vi "加标回收启动对话框.vi"(11 "测试模式":enum16{"水样测试", "平行样测试", "加标回收", "集成干预测试"}(ring)) -> (1 "流程参数":T2, 2 "启动参数":T3, 3 "check ？":bool)   [LabVIEW 2016, in "质控单元V2.lvlib"]
panel:
  in  "静态加标设置":T1
  in  "采配水":bool=TRUE
  in  "取消":bool
  in  "确认":bool
  in  "CODCr":bool caption="启用"
  in  "CODMn":bool caption="启用"
  in  "总氮":bool caption="启用"
  in  "总磷":bool caption="启用"
  in  "氨氮":bool caption="启用"
  # "请选择启动参数和流程"
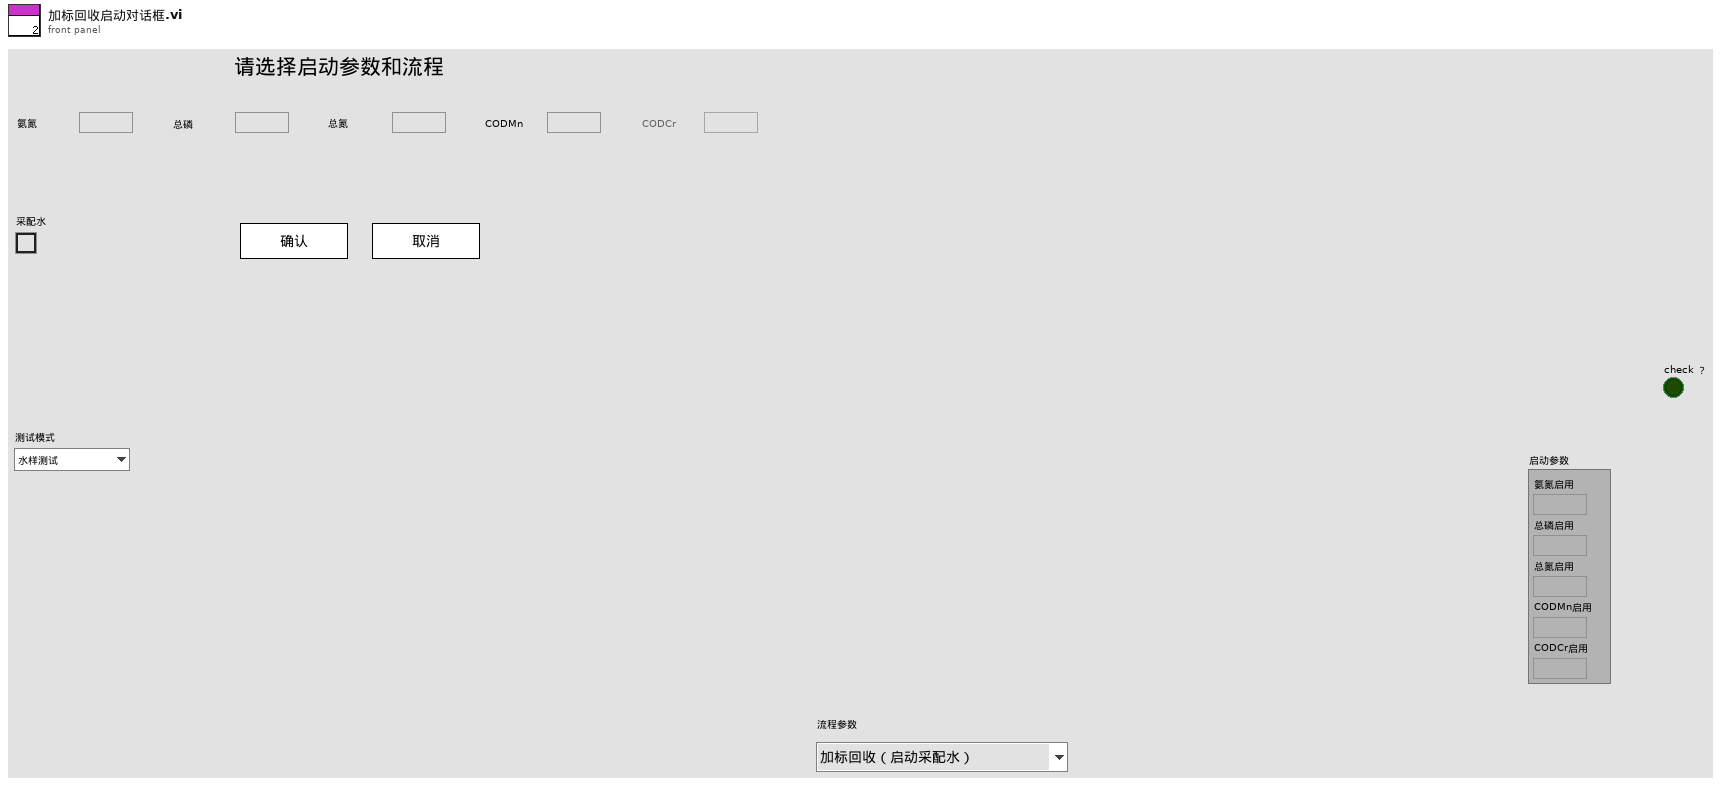
[diagram p1: front panel]
types:
  T1 = cluster{"氨氮静态加标":cluster{"静态加标：":bool, "加标体积":sgl}, "总磷静态加标":cluster{"静态加标：":bool, "加标体积":sgl}, "总氮静态加标":cluster{"静态加标：":bool, "加标体积":sgl}, "CODMn静态加标":cluster{"静态加标：":bool, "加标体积":sgl}, "CODCr静态加标":cluster{"静态加标：":bool, "加标体积":sgl}, "氟化物静态加标":cluster{"静态加标：":bool, "加标体积":sgl}, "挥发酚静态加标":cluster{"静态加标：":bool, "加标体积":sgl}}
  T2 = typedef "质控单元V4.lvlib/测试流程.ctl" = enum16{"加标回收（启动采配水）", "加标回收（不启动采配水）", "水样测试（启动采配水）", "水样测试（不启动采配水）", "平行样测试（启动采配水）", "平行样测试（不启动采配水）", "集成干预测试"}
  T3 = typedef "质控单元V2.lvlib/启动参数.ctl" = cluster{"氨氮启用":bool, "总磷启用":bool, "总氮启用":bool, "CODMn启用":bool, "CODCr启用":bool}
  T4 = cluster{"氨氮":bool, "总磷":bool, "总氮":bool, "CODMn":bool, "CODCr":bool, "氨氮总磷":bool, "总磷总氮":bool}
  T5 = typedef "质控单元V2.lvlib/测试流程.ctl" = enum16{"加标回收（启动采配水）", "加标回收（不启动采配水）", "水样测试（启动采配水）", "水样测试（不启动采配水）", "平行样测试（启动采配水）", "平行样测试（不启动采配水）", "集成干预测试"}
  T6 = cluster{"氨氮":bool, "总磷":bool, "总氮":bool, "CODMn":bool, "CODCr":bool}
  T7 = enum8{"Enabled", "Disabled", "Disabled and Grayed Out"}
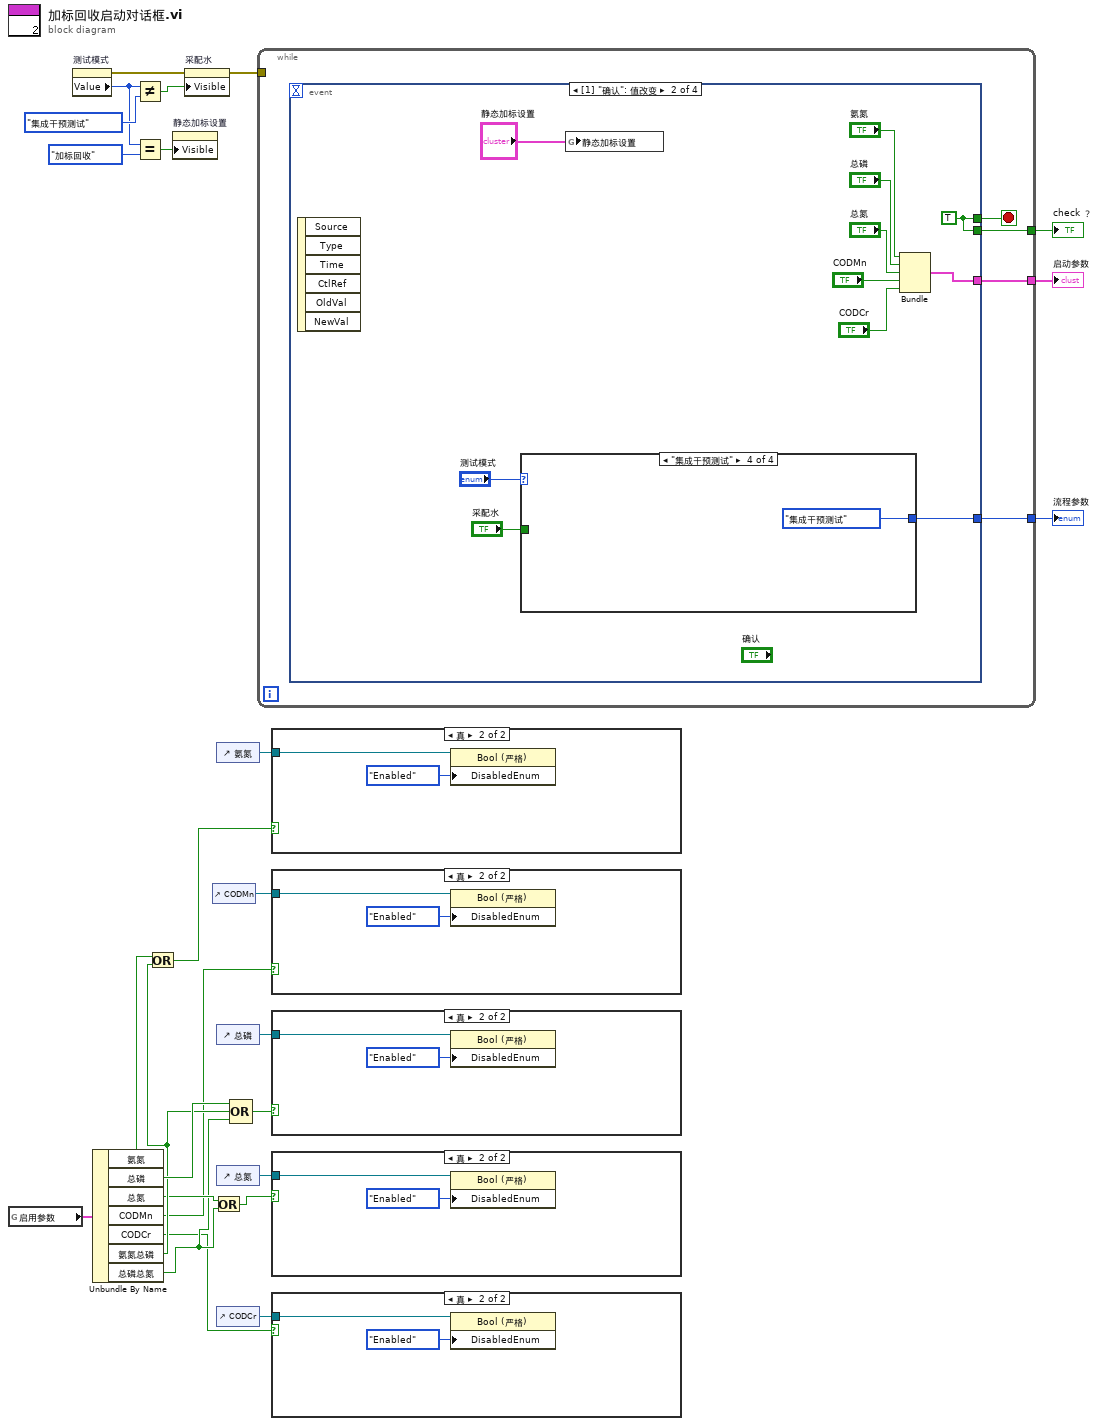
[diagram p0: block diagram]
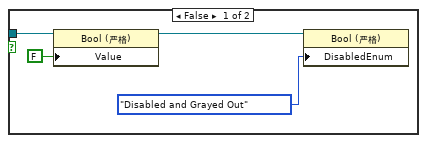
[diagram p2: hidden frame]
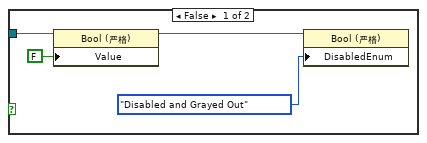
[diagram p3: hidden frame]
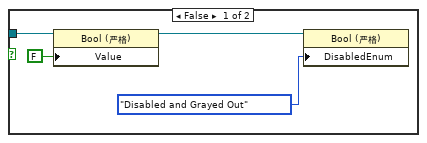
[diagram p4: hidden frame]
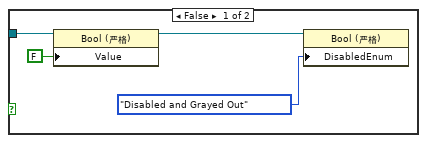
[diagram p5: hidden frame]
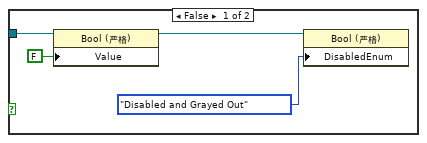
[diagram p6: hidden frame]
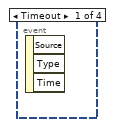
[diagram p7: hidden frame]
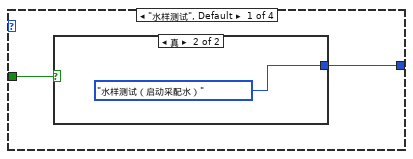
[diagram p8: hidden frame]
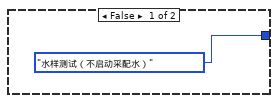
[diagram p9: hidden frame]
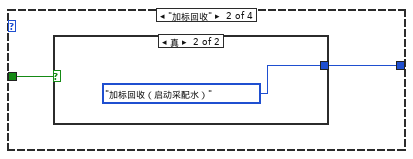
[diagram p10: hidden frame]
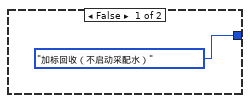
[diagram p11: hidden frame]
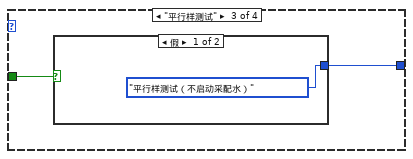
[diagram p12: hidden frame]
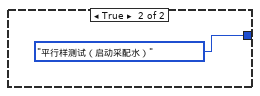
[diagram p13: hidden frame]
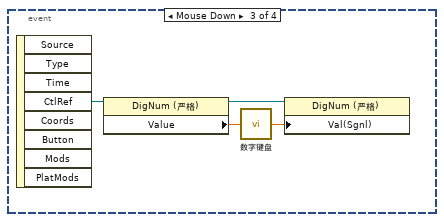
[diagram p14: hidden frame]
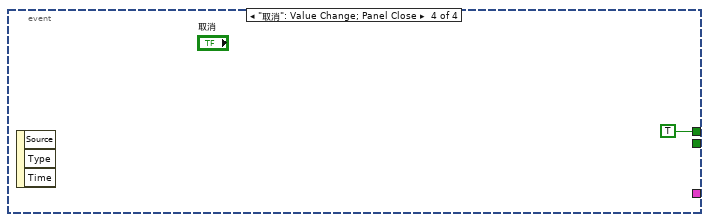
[diagram p15: hidden frame]
diagram:
  n1 = global read "ZK断电保存全局变量.vi" "启用参数"() -> (w18:T4)
  n2 = property on="测试模式" class="Enum (严格)"() -> (error out=w16:errorcluster, "Value"=w13:enum16{"水样测试", "平行样测试", "加标回收", "集成干预测试"})  [unwired: 2 in, 1 out]
  n3 = Unbundle By Name(w18) -> ("氨氮"=w10:bool, "总磷"=w8:bool, "总氮"=w5:bool, "CODMn"=w1:bool, "CODCr"=w2:bool, "氨氮总磷"=w7:bool, "总磷总氮"=w4:bool)
  n4 = Not Equal?(x=w13, y=enum16{"水样测试", "平行样测试", "加标回收", "集成干预测试"}."集成干预测试") -> (x != y?=w15:bool)
  n5 = Equal?(x=w13, y=enum16{"水样测试", "平行样测试", "加标回收", "集成干预测试"}."加标回收") -> (x = y?=w11:bool)
  n6 = Or(x=w10, y=w7) -> (x .or. y?=w9:bool)
  n7 = property on="静态加标设置" class="Clust (严格)"("Visible"=w11) -> ()  [unwired: 2 in, 2 out]
  n8 = property on="采配水" class="Bool (严格)"(error in=w16, "Visible"=w15) -> (error out=w14:errorcluster)  [unwired: 1 in, 1 out]
  n9 = control-ref of="CODMn"() -> (w20:refnum<vi>)
  n10 = Or(x=w5, y=w4) -> (x .or. y?=w3:bool)
  n11 = control-ref of="氨氮"() -> (w23:refnum<vi>)
  n12 = control-ref of="总磷"() -> (w22:refnum<vi>)
  n13 = control-ref of="总氮"() -> (w21:refnum<vi>)
  n14 = control-ref of="CODCr"() -> (w19:refnum<vi>)
  n15 = Compound Arithmetic op=OR ("复合运算")(w8, w7, w4) -> (w6:bool)
  n16 = while {
    tunnel: [w30] -> w26
    tunnel: [w28] -> w25
    tunnel: [w27] -> w24
    tunnel: w14 -> [_]
    stop <- w29 stop-if-true
    n17 = event shown="[1] \"确认\": 值改变" {
      selector: _ -> [_ _ _ _]
      dyn-events: _ -> [_ _ _ _]
      timeout: _ -> [_ _ _ _]
      tunnel: [_ w41 _ _] -> w30
      tunnel: [_ w41 _ TRUE] -> w29
      tunnel: [_ w35 _ _] -> w28
      tunnel: [_ w33 _ _] -> w27
      event Timeout {
        n18 = event-data() -> ()  [unwired: 1 in, 3 out]
      }
      event "确认": Value Change {
        w41 = TRUE
        n19 = event-data() -> ()  [unwired: 1 in, 6 out]
        n20 = case shown="\"集成干预测试\"" "测试模式" {
          tunnel: "采配水" -> [w43 w47 w51 _]
          tunnel: [w42 w46 w50 测试流程."集成干预测试" ("流程")] -> w33
          frame "水样测试", Default {
            n21 = case shown="真" w43 {
              tunnel: [测试流程."水样测试（不启动采配水）" ("流程") 测试流程."水样测试（启动采配水）" ("流程")] -> w42
              frame False {
              }
              frame True {
              }
            }
          }
          frame "加标回收" {
            n22 = case shown="真" w47 {
              tunnel: [测试流程."加标回收（不启动采配水）" ("流程") 测试流程."加标回收（启动采配水）" ("流程")] -> w46
              frame False {
              }
              frame True {
              }
            }
          }
          frame "平行样测试" {
            n23 = case shown="假" w51 {
              tunnel: [测试流程."平行样测试（不启动采配水）" ("流程") 测试流程."平行样测试（启动采配水）" ("流程")] -> w50
              frame False {
              }
              frame True {
              }
            }
          }
          frame "集成干预测试" {
          }
        }
        n24 = global write "ZK非断电保存全局变量.vi" "静态加标设置"("静态加标设置") -> ()
        n25 = Bundle("氨氮"="氨氮", "总磷"="总磷", "总氮"="总氮", "CODMn"="CODMn", "CODCr"="CODCr") -> (w35:T6)  [unwired: 1 in]
      }
      event "静态加标设置.氨氮静态加标.加标体积", "静态加标设置.总磷静态加标.加标体积", "静态加标设置.总氮静态加标.加标体积", "静态加标设置.CODMn静态加标.加标体积", "静态加标设置.CODCr静态加标.加标体积", "静态加标设置.氟化物静态加标.加标体积", "静态加标设置.挥发酚静态加标.加标体积": Mouse Down {
        n26 = event-data() -> ("CtlRef"=w55:refnum<vi>)  [unwired: 1 in, 7 out]
        n27 = property class="DigNum (严格)"(reference=w55) -> (reference out=w58:refnum<vi>, "Value"=w56:sgl)  [unwired: 1 in, 1 out]
        n28 = call "数字键盘.vi"("OldNumber"=w56) -> ("NewNumber"=w57:sgl)
        n29 = property class="DigNum (严格)"(reference=w58, "Val(Sgnl)"=w57) -> ()  [unwired: 1 in, 2 out]
      }
      event "取消": Value Change; Panel Close {
        n30 = event-data() -> ()  [unwired: 1 in, 3 out]
      }
    }
  }
  "check ？" <- w26
  "启动参数" <- w25
  "流程参数" <- w24
  n31 = case shown="真" w9 {
    tunnel: w23 -> [w63 w64]
    frame False {
      n32 = property class="Bool (严格)"(reference=w63, "Value"=FALSE ("值")) -> (reference out=w61:refnum<vi>)  [unwired: 1 in, 1 out]
      n33 = property class="Bool (严格)"(reference=w61, "DisabledEnum"=T7."Disabled and Grayed Out" ("禁用")) -> ()  [unwired: 1 in, 2 out]
    }
    frame True {
      n34 = property class="Bool (严格)"(reference=w64, "DisabledEnum"=T7."Enabled" ("禁用")) -> ()  [unwired: 1 in, 2 out]
    }
  }
  n35 = case shown="真" w1 {
    tunnel: w20 -> [w69 w70]
    frame False {
      n36 = property class="Bool (严格)"(reference=w69, "Value"=FALSE ("值")) -> (reference out=w67:refnum<vi>)  [unwired: 1 in, 1 out]
      n37 = property class="Bool (严格)"(reference=w67, "DisabledEnum"=T7."Disabled and Grayed Out" ("禁用")) -> ()  [unwired: 1 in, 2 out]
    }
    frame True {
      n38 = property class="Bool (严格)"(reference=w70, "DisabledEnum"=T7."Enabled" ("禁用")) -> ()  [unwired: 1 in, 2 out]
    }
  }
  n39 = case shown="真" w6 {
    tunnel: w22 -> [w75 w76]
    frame False {
      n40 = property class="Bool (严格)"(reference=w75, "Value"=FALSE ("值")) -> (reference out=w73:refnum<vi>)  [unwired: 1 in, 1 out]
      n41 = property class="Bool (严格)"(reference=w73, "DisabledEnum"=T7."Disabled and Grayed Out" ("禁用")) -> ()  [unwired: 1 in, 2 out]
    }
    frame True {
      n42 = property class="Bool (严格)"(reference=w76, "DisabledEnum"=T7."Enabled" ("禁用")) -> ()  [unwired: 1 in, 2 out]
    }
  }
  n43 = case shown="真" w3 {
    tunnel: w21 -> [w81 w82]
    frame False {
      n44 = property class="Bool (严格)"(reference=w81, "Value"=FALSE ("值")) -> (reference out=w79:refnum<vi>)  [unwired: 1 in, 1 out]
      n45 = property class="Bool (严格)"(reference=w79, "DisabledEnum"=T7."Disabled and Grayed Out" ("禁用")) -> ()  [unwired: 1 in, 2 out]
    }
    frame True {
      n46 = property class="Bool (严格)"(reference=w82, "DisabledEnum"=T7."Enabled" ("禁用")) -> ()  [unwired: 1 in, 2 out]
    }
  }
  n47 = case shown="真" w2 {
    tunnel: w19 -> [w87 w88]
    frame False {
      n48 = property class="Bool (严格)"(reference=w87, "Value"=FALSE ("值")) -> (reference out=w85:refnum<vi>)  [unwired: 1 in, 1 out]
      n49 = property class="Bool (严格)"(reference=w85, "DisabledEnum"=T7."Disabled and Grayed Out" ("禁用")) -> ()  [unwired: 1 in, 2 out]
    }
    frame True {
      n50 = property class="Bool (严格)"(reference=w88, "DisabledEnum"=T7."Enabled" ("禁用")) -> ()  [unwired: 1 in, 2 out]
    }
  }
